vi "Launcher.vi"(8 "error in (no error)":errorcluster, 11 "Assembler in":refnum<class "Assembler.lvclass">) -> (0 "error out":errorcluster, 3 "Assembler out":refnum<class "Assembler.lvclass">)   [LabVIEW 2019, in "TimingDRV Engine.lvlib" / "Assembler.lvclass"]
uses:
  Assembler.lvclass
  Assembler.lvclass/Assembler.ctl
  Parent Classes/Process/Process.lvclass/Process.ctl
  Parent Classes/Process/Process.lvclass
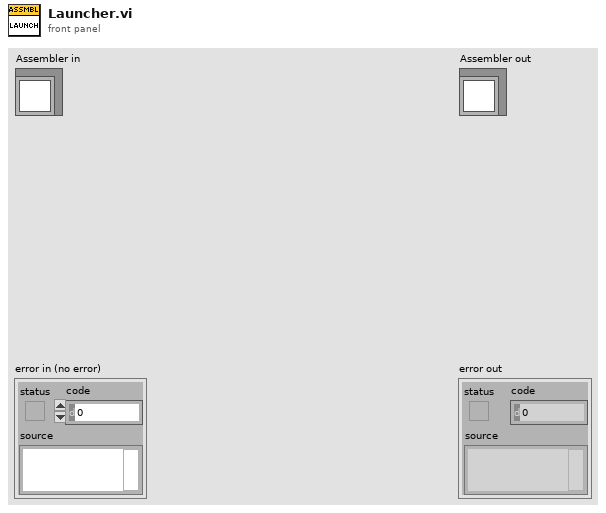
[diagram p1: front panel]
types:
  T1 = typedef "TimingDRV Engine.lvlib/Assembler.lvclass/Process Configuration.ctl" = cluster{"Process Timeout":dbl}
  T2 = typedef "TimingDRV Engine.lvlib/Process.lvclass/Process Lookup.ctl" = cluster{"Process ID":string, "MessageQ":refnum<queue>, "Update UE":refnum<user-event>}
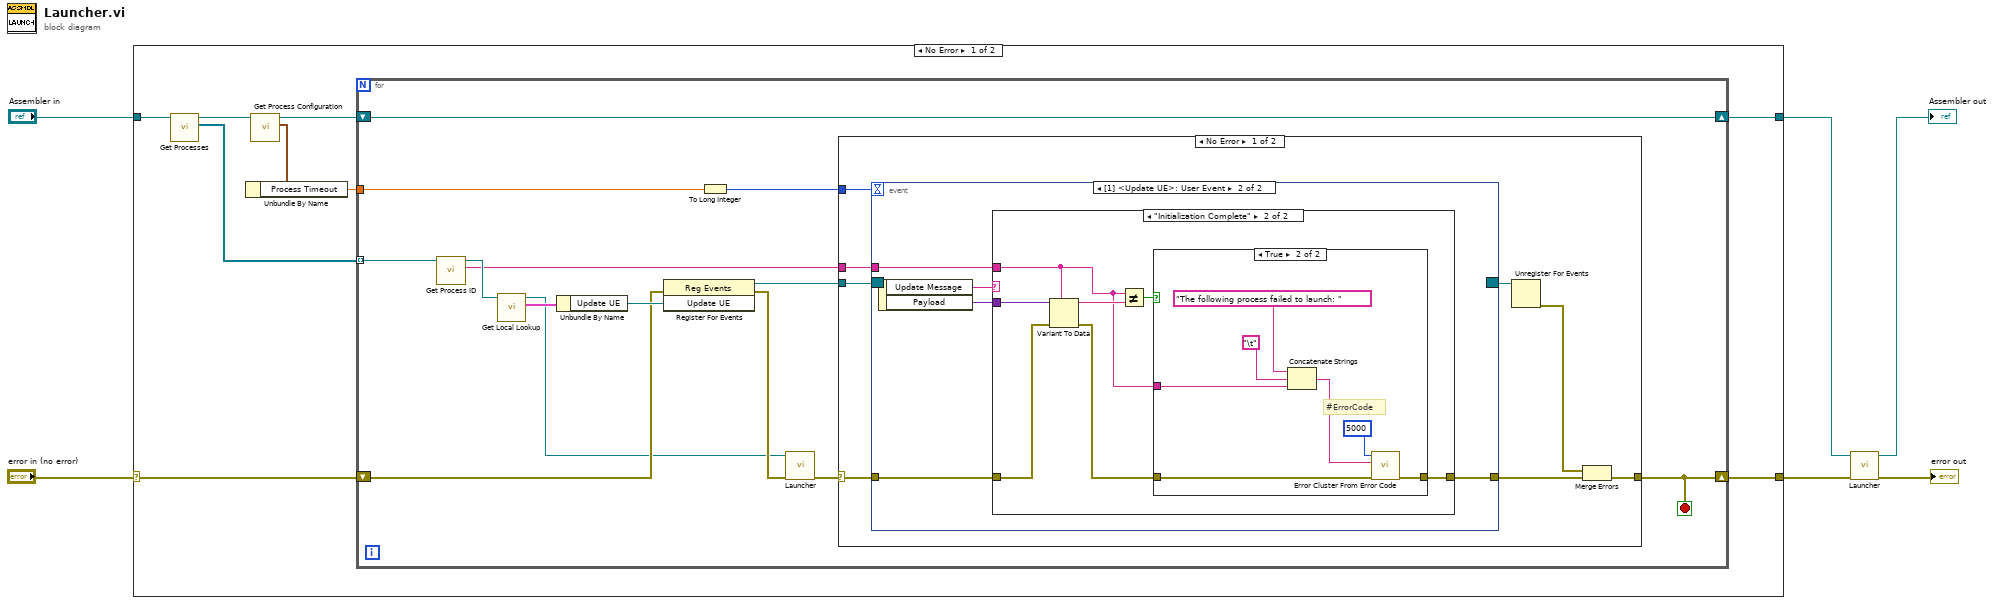
[diagram p0: block diagram]
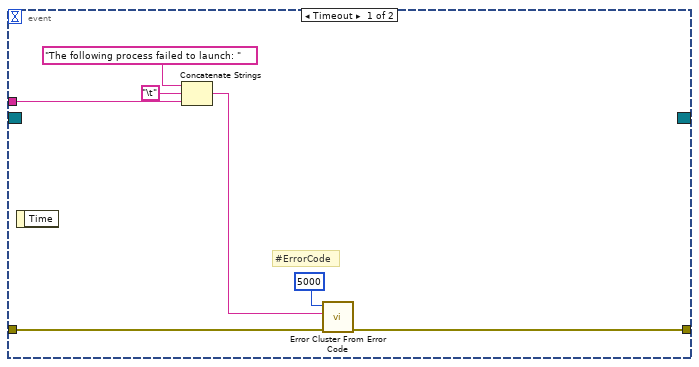
[diagram p2: hidden frame]
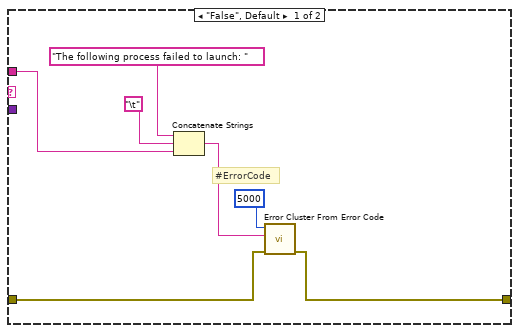
[diagram p3: hidden frame]
diagram:
  n1 = case shown="No Error" "error in (no error)" {
    selector: "error in (no error)" -> [w13 w74]
    tunnel: "Assembler in" -> [w14 w73]
    tunnel: [w8 w73] -> w4
    tunnel: [w7 w74] -> w1
    frame No Error {
      n2 = call "Get Processes.vi"("Assembler in"=w14) -> ("Processes"=w15:refnum<class "Process.lvclass">[], "Assembler out"=w12:refnum<class "Assembler.lvclass">)  [unwired: 9 in]
      n3 = call "Get Process Configuration.vi"("Assembler in"=w12) -> ("Process Settings"=w10:T1, "Assembler out"=w11:refnum<class "Assembler.lvclass">)  [unwired: 9 in]
      n4 = Unbundle By Name(w10) -> ("Process Timeout"=w9:dbl)
      n5 = for {
        tunnel: w15 -> [w24] mode=indexing
        shift-right: [w17] -> w8
        shift-left: w11 -> [w17]
        shift-right: [w20] -> w7
        shift-left: w13 -> [w22]
        tunnel: w9 -> [w19]
        stop <- w20 stop-if-true
        n6 = call "Get Process ID.vi"("CD_Process in"=w24) -> ("Process ID"=w21:string, "CD_Process out"=w23:refnum<class "Process.lvclass">)  [unwired: 9 in]
        n7 = call-dynamic "Get Local Lookup.vi"("Process in"=w23) -> ("Process Lookup"=w29:T2, "Process out"=w18:refnum<class "Process.lvclass">)  [unwired: 8 in, 1 out]
        n8 = Unbundle By Name(w29) -> ("Update UE"=w28:refnum<user-event>)
        n9 = register-events(error in=w22, w28) -> (reference out=w27:refnum<event-registration>, error out=w25:errorcluster)  [unwired: 1 in]
        n10 = To Long Integer(number=w19) -> (32bit integer=w26:i32)
        n11 = call-dynamic "Launcher.vi"("error in (no error)"=w25, "Process in"=w18) -> ("error out"=w16:errorcluster)  [unwired: 8 in, 1 out]
        n12 = case shown="No Error" w16 {
          selector: w16 -> [w30 w72]
          tunnel: w27 -> [w37 _]
          tunnel: w26 -> [w36 _]
          tunnel: w21 -> [w34 _]
          tunnel: [w31 w72] -> w20
          frame No Error {
            n13 = event shown="[1] <Update UE>: User Event" {
              selector: w37 -> [_ _]
              dyn-events: [_ _] -> w35
              timeout: w36 -> [_ _]
              tunnel: w34 -> [w42 w45]
              tunnel: w30 -> [w40 w47]
              tunnel: [w39 w46] -> w33
              event Timeout {
                # "#ErrorCode"
                n14 = event-data() -> ()  [unwired: 1 in, 1 out]
                n15 = Concatenate Strings("The following process failed to launch: " ("string"), "\t", w42) -> (w41:string)
                n16 = call <vilib>:"Error Cluster From Error Code.vi"("error in (no error)"=w40, "error message (\"\")"=w41, "error code (0)"=5000) -> ("error out"=w39:errorcluster)  [unwired: 6 in]
              }
              event User Event {
                n17 = event-data() -> ("Update Message"=w49:string, "Payload"=w48:variant)  [unwired: 1 in]
                n18 = case shown="\"Initialization Complete\"" w49 {
                  tunnel: w48 -> [_ w63]
                  tunnel: w47 -> [w52 w62]
                  tunnel: [w51 w60] -> w46
                  tunnel: w45 -> [w50 w58]
                  frame "False", Default {
                    # "#ErrorCode"
                    n19 = Concatenate Strings("The following process failed to launch: " ("string"), "\t", w50) -> (w56:string)
                    n20 = call <vilib>:"Error Cluster From Error Code.vi"("error in (no error)"=w52, "error message (\"\")"=w56, "error code (0)"=5000) -> ("error out"=w51:errorcluster)  [unwired: 6 in]
                  }
                  frame "Initialization Complete" {
                    n21 = Variant To Data(error in=w62, type=w58, Variant=w63) -> (data=w59:string, error out=w61:errorcluster)
                    n22 = Not Equal?(x=w58, y=w59) -> (x != y?=w57:bool)
                    n23 = case shown="True" w57 {
                      tunnel: w61 -> [w64 w67]
                      tunnel: [w64 w66] -> w60
                      tunnel: w58 -> [_ w65]
                      frame False {
                      }
                      frame True {
                        # "#ErrorCode"
                        n24 = Concatenate Strings("The following process failed to launch: " ("string"), "\t", w65) -> (w71:string)
                        n25 = call <vilib>:"Error Cluster From Error Code.vi"("error in (no error)"=w67, "error message (\"\")"=w71, "error code (0)"=5000) -> ("error out"=w66:errorcluster)  [unwired: 6 in]
                      }
                    }
                  }
                }
              }
            }
            n26 = Unregister For Events(event registration refnum=w35) -> (error out=w32:errorcluster)  [unwired: 1 in]
            n27 = Merge Errors(w32, w33) -> (w31:errorcluster)
          }
          frame Error {
          }
        }
      }
    }
    frame Error {
    }
  }
  n28 = call-parent "Launcher.vi"("error in (no error)"=w1, "Process in"=w4) -> ("error out"=→"error out":errorcluster, "Process out"=→"Assembler out":refnum<class "Assembler.lvclass">)  [unwired: 8 in]
